vi "Read Frequency Counter.vi"(8 "error in (no error)":errorcluster, 11 "VISA resource name":refnum<visa-resource-name>) -> (0 "error out":errorcluster, 1 "Positive Width":dbl, 2 "Duty":dbl, 3 "VISA resource name out":refnum<visa-resource-name>, 4 "Negative Width":dbl, 5 "Frequency":dbl, 6 "Frequency Deviation":dbl format="%#_6e")   [LabVIEW 2015, in "SDG X Series.lvlib"]
doc: "Reads the frequency, duty, positive width, negative width and frequency deviation from the frequency counter.\n\nNote: \n\nFrequency counter must be enabled first before running this vi. Use <b>Configure Frequency Counter.vi</b> to enable it."
uses:
  <instrlib>/SDG X Series/SDG X Series.lvlib
panel:
  # "Hz"
  # "%"
  # "s"
  # "s"
  # "ppm"
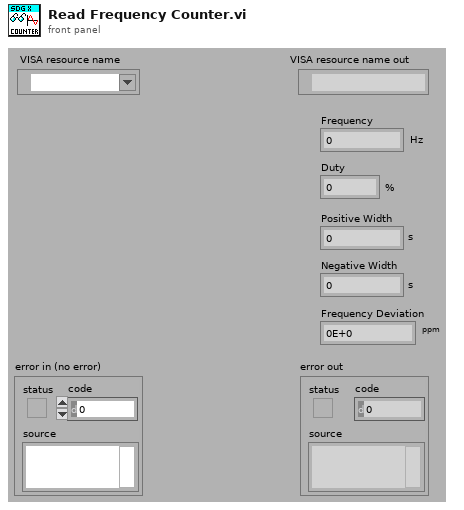
[diagram p1: front panel]
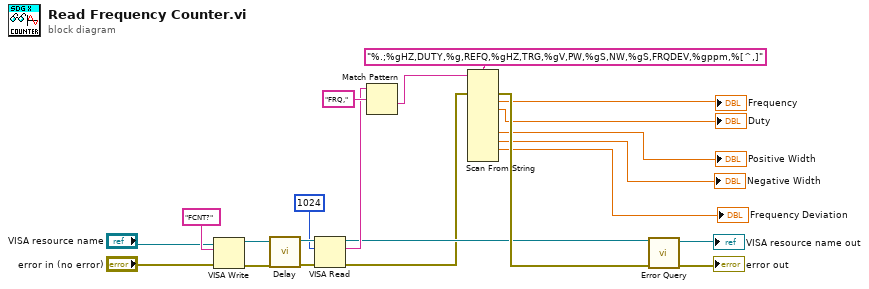
[diagram p0: block diagram]
diagram:
  n1 = VISA Write(VISA resource name="VISA resource name", write buffer="FCNT?", error in (no error)="error in (no error)") -> (VISA resource name out=w21:refnum<visa-resource-name>, error out=w20:errorcluster)  [unwired: 1 out]
  n2 = call <instrlib>:"Delay.vi"("error in (no error)"=w20, "VISA resource name"=w21) -> ("error out"=w7:errorcluster, "VISA resource name out"=w6:refnum<visa-resource-name>)  [unwired: 8 in]
  n3 = VISA Read(VISA resource name=w6, byte count=u32 1024 ("字节总数"), error in (no error)=w7) -> (VISA resource name out=w4:refnum<visa-resource-name>, read buffer=w5:string, error out=w3:errorcluster)  [unwired: 1 out]
  n4 = Match Pattern(string=w5, regular expression="FRQ,") -> (after substring=w11:string)  [unwired: 1 in, 3 out]
  n5 = Scan From String(format string="%.;%gHZ,DUTY,%g,REFQ,%gHZ,TRG,%gV,PW,%gS,NW,%gS,FRQDEV,%gppm,%[^,]", input string=w11, error in=w3) -> (error out=w17:errorcluster, output 1=→"Frequency":dbl, output 2=→"Duty":dbl, output 5=→"Positive Width":dbl, output 6=→"Negative Width":dbl, output 7=→"Frequency Deviation":dbl)  [unwired: 12 in, 2 out]
  n6 = call <instrlib>:"Error Query.vi"("error in (no error)"=w17, "VISA resource name"=w4) -> ("error out"=→"error out":errorcluster, "VISA resource name out"=→"VISA resource name out":refnum<visa-resource-name>)  [unwired: 6 in, 2 out]
